vi "Cal74100.vi"() -> ()   [LabVIEW 2013]
uses:
  <vilib>/Instr/_visa.llb/VISA Configure Serial Port (Instr).vi
panel:
  out "Info":string
  in  "Zero 3":string
  in  "Zero 2":string
  in  "Zero 1":string
  in  "Set":bool
  in  "Wavelength":string
  in  "Filt6":bool
  in  "Filt5":bool
  in  "Filt4":bool
  in  "Filt3":bool
  in  "Filt2":bool
  in  "Filt1":bool
  in  "Grat3":bool
  in  "Grat2":bool
  in  "Port2":bool
  in  "Port1":bool
  in  "Grat1":bool
  in  "CloseS":bool
  in  "OpenS":bool
  in  "Filter 6":string="\r\n"
  in  "Filter 5":string
  in  "Filter 1":string="\r\n"
  in  "Filter 2":string
  in  "Filter 3":string
  in  "Filter 4":string
  in  "Write":bool
  in  "Exit":bool
  in  "Read":bool
  in  "Label 3":string
  in  "Lines 3":string
  in  "Factor 3":string
  in  "Offset 3":string
  in  "Label 2":string
  in  "Lines 2":string
  in  "Factor 2":string
  in  "Offset 2":string
  in  "Offset 1":string
  in  "Factor 1":string
  in  "Lines 1":string
  in  "Label 1":string
  out "Current Grating":string
  out "State":string
  in  "Monochromator":refnum<visa-resource-name>="COM5"
  out "Next State":string
  out "error":T1
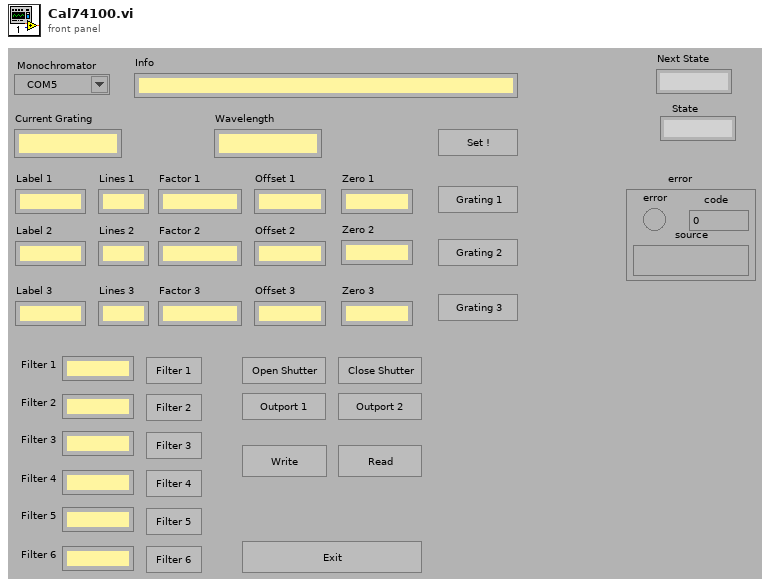
[diagram p1: front panel]
types:
  T1 = cluster{"error":bool, "code":i32, "source":string}
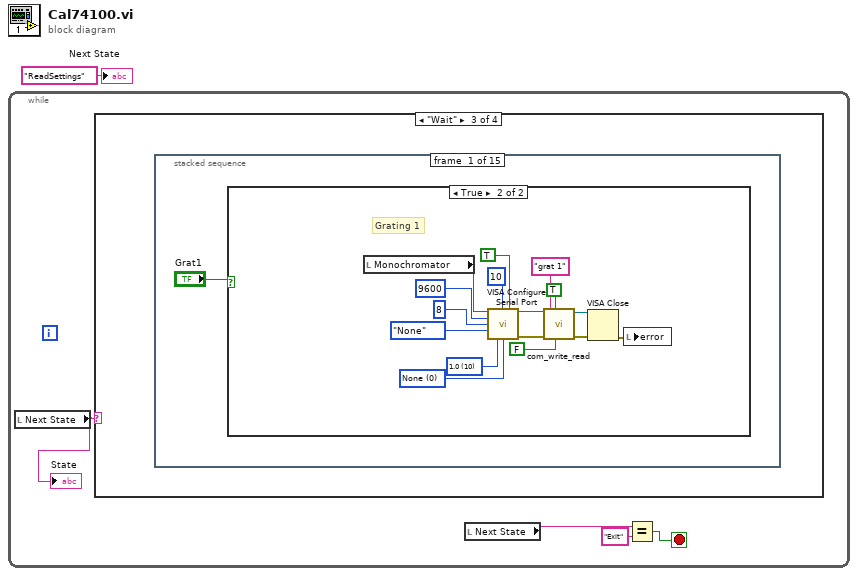
[diagram p0: block diagram]
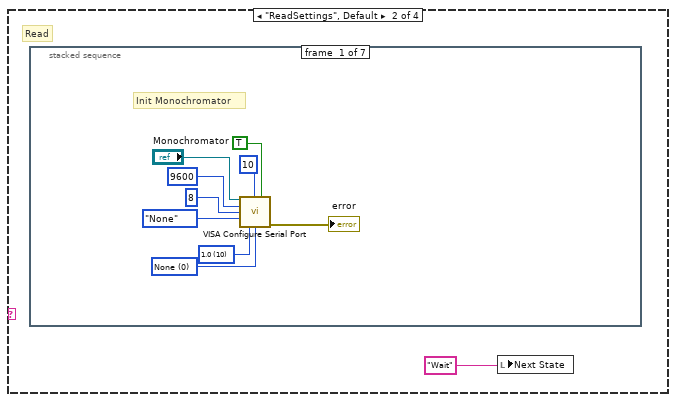
[diagram p3: hidden frame]
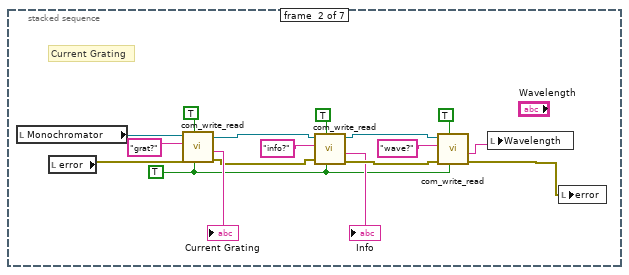
[diagram p4: hidden frame]
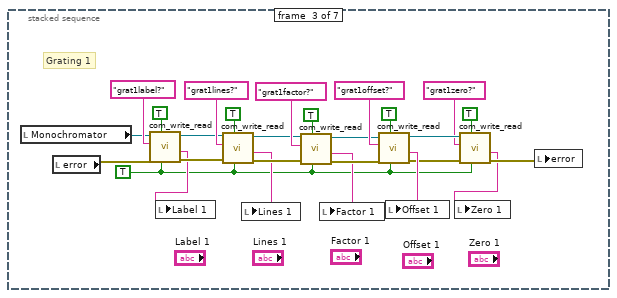
[diagram p5: hidden frame]
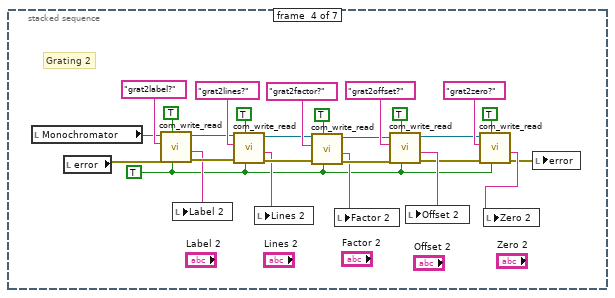
[diagram p6: hidden frame]
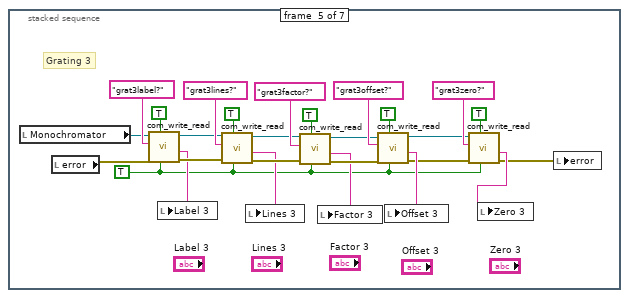
[diagram p7: hidden frame]
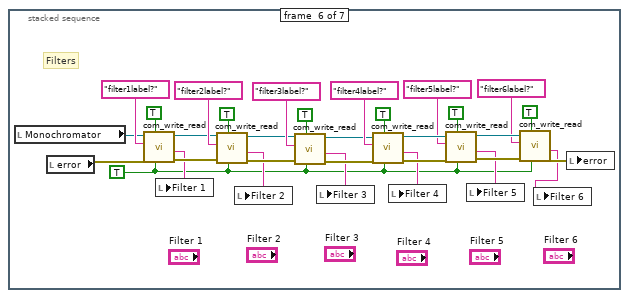
[diagram p8: hidden frame]
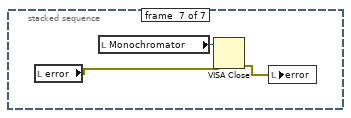
[diagram p9: hidden frame]
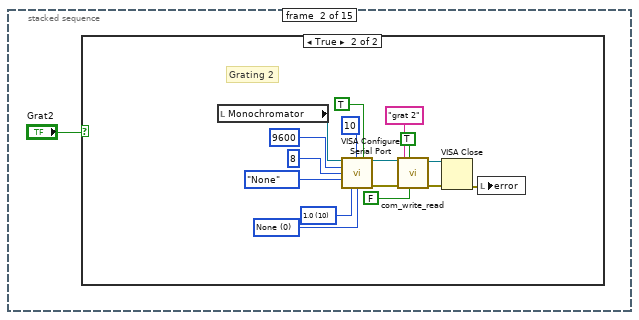
[diagram p11: hidden frame]
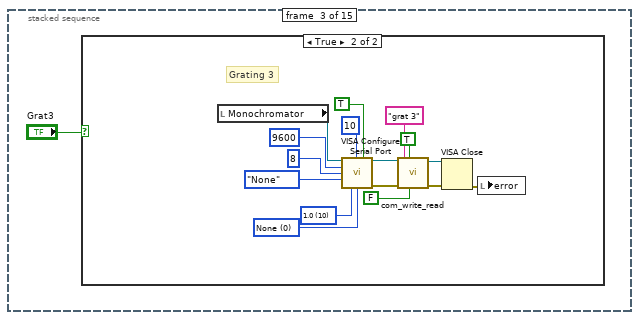
[diagram p13: hidden frame]
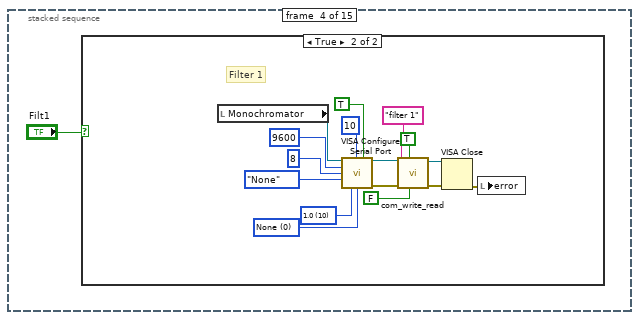
[diagram p15: hidden frame]
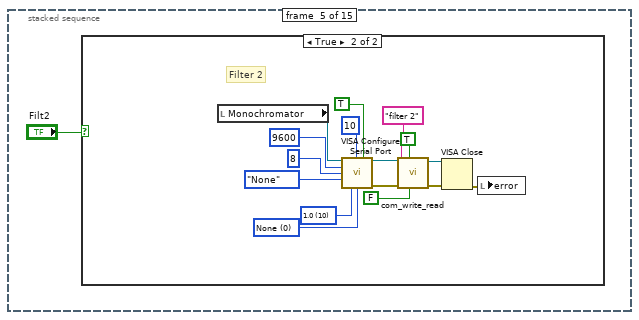
[diagram p17: hidden frame]
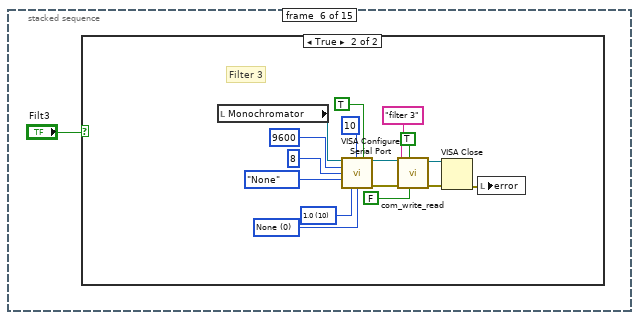
[diagram p19: hidden frame]
diagram:
  n1 = while {
    stop <- w4 stop-if-true
    n2 = local read "Next State"() -> (w2:string)
    "State" <- w2
    n3 = case shown="\"Wait\"" w2 {
      frame "Exit" {
      }
      frame "ReadSettings", Default {
        # "Read"
        n4 = stacked-sequence {
          frame #0 {
            w13 = u16 0 items=["None", "XON/XOFF", "RTS/CTS", "XON/XOFF & RTS/CTS", "DTR/DSR", "XON/XOFF & DTR/DSR"] ("flow control (0:none)")
            w12 = u16 10 items=["1.0"=10, "1.5"=15, "2.0"=20] ("stop bits (10: 1 bit)")
            # "Init Monochromator"
            n5 = call-poly "VISA Configure Serial Port"("VISA resource name"="Monochromator", "termination char\n(0xA = '\\n' = LF)"=u8 10 ("termination char\n(0xA = '\\n' = LF)"), "Enable Termination\nChar (T)"=TRUE, "baud rate (9600)"=u32 9600, "data bits (8)"=u16 8, "parity (0:none)"=enum16{"None", "Odd", "Even", "Mark", "Space"}."None", "stop bits (10: 1 bit)"=w12, "flow control (0:none)"=w13) -> ("error out"=→"error":errorcluster)  [unwired: 6 in, 1 out]
          }
          frame #1 {
            w16 = TRUE ("2 nd Query?")
            # "Current Grating"
            n6 = local read "Monochromator"() -> (w29:refnum<visa-resource-name>)
            n7 = local read "error"() -> (w30:T1)
            n8 = call "com_write_read.vi"("2 nd Query?"=w16, "Query?"=TRUE, "error in"=w30, "Command"="grat?" ("write buffer"), "VISA handle in"=w29) -> ("error out"=w21:errorcluster, "2nd Response"=→"Current Grating":string, "VISA handle out"=w20:refnum<visa-resource-name>)  [unwired: 1 in, 2 out]
            n9 = call "com_write_read.vi"("2 nd Query?"=w16, "Query?"=TRUE, "error in"=w21, "Command"="info?" ("write buffer"), "VISA handle in"=w20) -> ("error out"=w18:errorcluster, "2nd Response"=→"Info":string, "VISA handle out"=w19:refnum<visa-resource-name>)  [unwired: 1 in, 2 out]
            n10 = call "com_write_read.vi"("2 nd Query?"=w16, "Query?"=TRUE, "error in"=w18, "Command"="wave?" ("write buffer"), "VISA handle in"=w19) -> ("error out"=w26:errorcluster, "2nd Response"=w24:string)  [unwired: 1 in, 3 out]
            n11 = local write "Wavelength"(w24) -> ()
            n12 = local write "error"(w26) -> ()
          }
          frame #2 {
            w33 = TRUE ("2 nd Query?")
            # "Grating 1"
            n13 = local read "Monochromator"() -> (w56:refnum<visa-resource-name>)
            n14 = local read "error"() -> (w57:T1)
            n15 = call "com_write_read.vi"("2 nd Query?"=w33, "Query?"=TRUE, "error in"=w57, "Command"="grat1label?" ("write buffer"), "VISA handle in"=w56) -> ("error out"=w46:errorcluster, "2nd Response"=w43:string, "VISA handle out"=w49:refnum<visa-resource-name>)  [unwired: 1 in, 2 out]
            n16 = local write "Label 1"(w43) -> ()
            n17 = call "com_write_read.vi"("2 nd Query?"=w33, "Query?"=TRUE, "error in"=w46, "Command"="grat1lines?" ("write buffer"), "VISA handle in"=w49) -> ("error out"=w45:errorcluster, "2nd Response"=w42:string, "VISA handle out"=w48:refnum<visa-resource-name>)  [unwired: 1 in, 2 out]
            n18 = local write "Lines 1"(w42) -> ()
            n19 = call "com_write_read.vi"("2 nd Query?"=w33, "Query?"=TRUE, "error in"=w45, "Command"="grat1factor?" ("write buffer"), "VISA handle in"=w48) -> ("error out"=w44:errorcluster, "2nd Response"=w41:string, "VISA handle out"=w47:refnum<visa-resource-name>)  [unwired: 1 in, 2 out]
            n20 = local write "Factor 1"(w41) -> ()
            n21 = call "com_write_read.vi"("2 nd Query?"=w33, "Query?"=TRUE, "error in"=w44, "Command"="grat1offset?" ("write buffer"), "VISA handle in"=w47) -> ("error out"=w37:errorcluster, "2nd Response"=w40:string, "VISA handle out"=w38:refnum<visa-resource-name>)  [unwired: 1 in, 2 out]
            n22 = local write "Offset 1"(w40) -> ()
            n23 = call "com_write_read.vi"("2 nd Query?"=w33, "Query?"=TRUE, "error in"=w37, "Command"="grat1zero?" ("write buffer"), "VISA handle in"=w38) -> ("error out"=w36:errorcluster, "2nd Response"=w35:string)  [unwired: 1 in, 3 out]
            n24 = local write "Zero 1"(w35) -> ()
            n25 = local write "error"(w36) -> ()
          }
          frame #3 {
            w60 = TRUE ("2 nd Query?")
            # "Grating 2"
            n26 = local read "Monochromator"() -> (w83:refnum<visa-resource-name>)
            n27 = local read "error"() -> (w84:T1)
            n28 = call "com_write_read.vi"("2 nd Query?"=w60, "Query?"=TRUE, "error in"=w84, "Command"="grat2label?" ("write buffer"), "VISA handle in"=w83) -> ("error out"=w73:errorcluster, "2nd Response"=w70:string, "VISA handle out"=w76:refnum<visa-resource-name>)  [unwired: 1 in, 2 out]
            n29 = local write "Label 2"(w70) -> ()
            n30 = call "com_write_read.vi"("2 nd Query?"=w60, "Query?"=TRUE, "error in"=w73, "Command"="grat2lines?" ("write buffer"), "VISA handle in"=w76) -> ("error out"=w72:errorcluster, "2nd Response"=w69:string, "VISA handle out"=w75:refnum<visa-resource-name>)  [unwired: 1 in, 2 out]
            n31 = local write "Lines 2"(w69) -> ()
            n32 = call "com_write_read.vi"("2 nd Query?"=w60, "Query?"=TRUE, "error in"=w72, "Command"="grat2factor?" ("write buffer"), "VISA handle in"=w75) -> ("error out"=w71:errorcluster, "2nd Response"=w68:string, "VISA handle out"=w74:refnum<visa-resource-name>)  [unwired: 1 in, 2 out]
            n33 = local write "Factor 2"(w68) -> ()
            n34 = call "com_write_read.vi"("2 nd Query?"=w60, "Query?"=TRUE, "error in"=w71, "Command"="grat2offset?" ("write buffer"), "VISA handle in"=w74) -> ("error out"=w63:errorcluster, "2nd Response"=w67:string, "VISA handle out"=w64:refnum<visa-resource-name>)  [unwired: 1 in, 2 out]
            n35 = local write "Offset 2"(w67) -> ()
            n36 = call "com_write_read.vi"("2 nd Query?"=w60, "Query?"=TRUE, "error in"=w63, "Command"="grat2zero?" ("write buffer"), "VISA handle in"=w64) -> ("error out"=w61:errorcluster, "2nd Response"=w62:string)  [unwired: 1 in, 3 out]
            n37 = local write "Zero 2"(w62) -> ()
            n38 = local write "error"(w61) -> ()
          }
          frame #4 {
            w87 = TRUE ("2 nd Query?")
            # "Grating 3"
            n39 = local read "Monochromator"() -> (w110:refnum<visa-resource-name>)
            n40 = local read "error"() -> (w111:T1)
            n41 = call "com_write_read.vi"("2 nd Query?"=w87, "Query?"=TRUE, "error in"=w111, "Command"="grat3label?" ("write buffer"), "VISA handle in"=w110) -> ("error out"=w100:errorcluster, "2nd Response"=w97:string, "VISA handle out"=w103:refnum<visa-resource-name>)  [unwired: 1 in, 2 out]
            n42 = local write "Label 3"(w97) -> ()
            n43 = call "com_write_read.vi"("2 nd Query?"=w87, "Query?"=TRUE, "error in"=w100, "Command"="grat3lines?" ("write buffer"), "VISA handle in"=w103) -> ("error out"=w99:errorcluster, "2nd Response"=w96:string, "VISA handle out"=w102:refnum<visa-resource-name>)  [unwired: 1 in, 2 out]
            n44 = local write "Lines 3"(w96) -> ()
            n45 = call "com_write_read.vi"("2 nd Query?"=w87, "Query?"=TRUE, "error in"=w99, "Command"="grat3factor?" ("write buffer"), "VISA handle in"=w102) -> ("error out"=w98:errorcluster, "2nd Response"=w95:string, "VISA handle out"=w101:refnum<visa-resource-name>)  [unwired: 1 in, 2 out]
            n46 = local write "Factor 3"(w95) -> ()
            n47 = call "com_write_read.vi"("2 nd Query?"=w87, "Query?"=TRUE, "error in"=w98, "Command"="grat3offset?" ("write buffer"), "VISA handle in"=w101) -> ("error out"=w90:errorcluster, "2nd Response"=w94:string, "VISA handle out"=w91:refnum<visa-resource-name>)  [unwired: 1 in, 2 out]
            n48 = local write "Offset 3"(w94) -> ()
            n49 = call "com_write_read.vi"("2 nd Query?"=w87, "Query?"=TRUE, "error in"=w90, "Command"="grat3zero?" ("write buffer"), "VISA handle in"=w91) -> ("error out"=w88:errorcluster, "2nd Response"=w89:string)  [unwired: 1 in, 3 out]
            n50 = local write "Zero 3"(w89) -> ()
            n51 = local write "error"(w88) -> ()
          }
          frame #5 {
            w114 = TRUE ("2 nd Query?")
            # "Filters"
            n52 = local read "Monochromator"() -> (w142:refnum<visa-resource-name>)
            n53 = local read "error"() -> (w143:T1)
            n54 = call "com_write_read.vi"("2 nd Query?"=w114, "Query?"=TRUE, "error in"=w143, "Command"="filter1label?" ("write buffer"), "VISA handle in"=w142) -> ("error out"=w132:errorcluster, "2nd Response"=w115:string, "VISA handle out"=w135:refnum<visa-resource-name>)  [unwired: 1 in, 2 out]
            n55 = local write "Filter 1"(w115) -> ()
            n56 = call "com_write_read.vi"("2 nd Query?"=w114, "Query?"=TRUE, "error in"=w132, "Command"="filter2label?" ("write buffer"), "VISA handle in"=w135) -> ("error out"=w131:errorcluster, "2nd Response"=w116:string, "VISA handle out"=w134:refnum<visa-resource-name>)  [unwired: 1 in, 2 out]
            n57 = local write "Filter 2"(w116) -> ()
            n58 = call "com_write_read.vi"("2 nd Query?"=w114, "Query?"=TRUE, "error in"=w131, "Command"="filter3label?" ("write buffer"), "VISA handle in"=w134) -> ("error out"=w130:errorcluster, "2nd Response"=w117:string, "VISA handle out"=w133:refnum<visa-resource-name>)  [unwired: 1 in, 2 out]
            n59 = local write "Filter 3"(w117) -> ()
            n60 = call "com_write_read.vi"("2 nd Query?"=w114, "Query?"=TRUE, "error in"=w130, "Command"="filter4label?" ("write buffer"), "VISA handle in"=w133) -> ("error out"=w127:errorcluster, "2nd Response"=w118:string, "VISA handle out"=w124:refnum<visa-resource-name>)  [unwired: 1 in, 2 out]
            n61 = local write "Filter 4"(w118) -> ()
            n62 = call "com_write_read.vi"("2 nd Query?"=w114, "Query?"=TRUE, "error in"=w127, "Command"="filter5label?" ("write buffer"), "VISA handle in"=w124) -> ("error out"=w126:errorcluster, "2nd Response"=w119:string, "VISA handle out"=w123:refnum<visa-resource-name>)  [unwired: 1 in, 2 out]
            n63 = local write "Filter 5"(w119) -> ()
            n64 = call "com_write_read.vi"("2 nd Query?"=w114, "Query?"=TRUE, "error in"=w126, "Command"="filter6label?" ("write buffer"), "VISA handle in"=w123) -> ("error out"=w125:errorcluster, "2nd Response"=w120:string)  [unwired: 1 in, 3 out]
            n65 = local write "Filter 6"(w120) -> ()
            n66 = local write "error"(w125) -> ()
          }
          frame #6 {
            n67 = local read "error"() -> (w146:T1)
            n68 = local read "Monochromator"() -> (w148:refnum<visa-resource-name>)
            n69 = VISA Close(VISA resource name=w148, error in (no error)=w146) -> (error out=w147:errorcluster)
            n70 = local write "error"(w147) -> ()
          }
        }
        n71 = local write "Next State"("Wait") -> ()
      }
      frame "Wait" {
        n72 = stacked-sequence {
          frame #0 {
            n73 = case shown="True" "Grat1" {
              frame False {
              }
              frame True {
                w153 = u16 0 items=["None", "XON/XOFF", "RTS/CTS", "XON/XOFF & RTS/CTS", "DTR/DSR", "XON/XOFF & DTR/DSR"] ("flow control (0:none)")
                w154 = u16 10 items=["1.0"=10, "1.5"=15, "2.0"=20] ("stop bits (10: 1 bit)")
                # "Grating 1"
                n74 = local read "Monochromator"() -> (w158:refnum<visa-resource-name>)
                n75 = call-poly "VISA Configure Serial Port"("VISA resource name"=w158, "termination char\n(0xA = '\\n' = LF)"=u8 10 ("termination char\n(0xA = '\\n' = LF)"), "Enable Termination\nChar (T)"=TRUE, "baud rate (9600)"=u32 9600, "data bits (8)"=u16 8, "parity (0:none)"=enum16{"None", "Odd", "Even", "Mark", "Space"}."None", "stop bits (10: 1 bit)"=w154, "flow control (0:none)"=w153) -> ("VISA resource name out"=w163:refnum<visa-resource-name>, "error out"=w162:errorcluster)  [unwired: 6 in]
                n76 = call "com_write_read.vi"("2 nd Query?"=FALSE, "Query?"=TRUE, "error in"=w162, "Command"="grat 1" ("write buffer"), "VISA handle in"=w163) -> ("error out"=w165:errorcluster, "VISA handle out"=w164:refnum<visa-resource-name>)  [unwired: 1 in, 3 out]
                n77 = VISA Close(VISA resource name=w164, error in (no error)=w165) -> (error out=w159:errorcluster)
                n78 = local write "error"(w159) -> ()
              }
            }
          }
          frame #1 {
            n79 = case shown="True" "Grat2" {
              frame False {
              }
              frame True {
                w170 = u16 0 items=["None", "XON/XOFF", "RTS/CTS", "XON/XOFF & RTS/CTS", "DTR/DSR", "XON/XOFF & DTR/DSR"] ("flow control (0:none)")
                w171 = u16 10 items=["1.0"=10, "1.5"=15, "2.0"=20] ("stop bits (10: 1 bit)")
                # "Grating 2"
                n80 = local read "Monochromator"() -> (w175:refnum<visa-resource-name>)
                n81 = call-poly "VISA Configure Serial Port"("VISA resource name"=w175, "termination char\n(0xA = '\\n' = LF)"=u8 10 ("termination char\n(0xA = '\\n' = LF)"), "Enable Termination\nChar (T)"=TRUE, "baud rate (9600)"=u32 9600, "data bits (8)"=u16 8, "parity (0:none)"=enum16{"None", "Odd", "Even", "Mark", "Space"}."None", "stop bits (10: 1 bit)"=w171, "flow control (0:none)"=w170) -> ("VISA resource name out"=w180:refnum<visa-resource-name>, "error out"=w179:errorcluster)  [unwired: 6 in]
                n82 = call "com_write_read.vi"("2 nd Query?"=FALSE, "Query?"=TRUE, "error in"=w179, "Command"="grat 2" ("write buffer"), "VISA handle in"=w180) -> ("error out"=w182:errorcluster, "VISA handle out"=w181:refnum<visa-resource-name>)  [unwired: 1 in, 3 out]
                n83 = VISA Close(VISA resource name=w181, error in (no error)=w182) -> (error out=w176:errorcluster)
                n84 = local write "error"(w176) -> ()
              }
            }
          }
          frame #2 {
            n85 = case shown="True" "Grat3" {
              frame False {
              }
              frame True {
                w187 = u16 0 items=["None", "XON/XOFF", "RTS/CTS", "XON/XOFF & RTS/CTS", "DTR/DSR", "XON/XOFF & DTR/DSR"] ("flow control (0:none)")
                w188 = u16 10 items=["1.0"=10, "1.5"=15, "2.0"=20] ("stop bits (10: 1 bit)")
                # "Grating 3"
                n86 = local read "Monochromator"() -> (w192:refnum<visa-resource-name>)
                n87 = call-poly "VISA Configure Serial Port"("VISA resource name"=w192, "termination char\n(0xA = '\\n' = LF)"=u8 10 ("termination char\n(0xA = '\\n' = LF)"), "Enable Termination\nChar (T)"=TRUE, "baud rate (9600)"=u32 9600, "data bits (8)"=u16 8, "parity (0:none)"=enum16{"None", "Odd", "Even", "Mark", "Space"}."None", "stop bits (10: 1 bit)"=w188, "flow control (0:none)"=w187) -> ("VISA resource name out"=w197:refnum<visa-resource-name>, "error out"=w196:errorcluster)  [unwired: 6 in]
                n88 = call "com_write_read.vi"("2 nd Query?"=FALSE, "Query?"=TRUE, "error in"=w196, "Command"="grat 3" ("write buffer"), "VISA handle in"=w197) -> ("error out"=w199:errorcluster, "VISA handle out"=w198:refnum<visa-resource-name>)  [unwired: 1 in, 3 out]
                n89 = VISA Close(VISA resource name=w198, error in (no error)=w199) -> (error out=w193:errorcluster)
                n90 = local write "error"(w193) -> ()
              }
            }
          }
          frame #3 {
            n91 = case shown="True" "Filt1" {
              frame False {
              }
              frame True {
                w204 = u16 0 items=["None", "XON/XOFF", "RTS/CTS", "XON/XOFF & RTS/CTS", "DTR/DSR", "XON/XOFF & DTR/DSR"] ("flow control (0:none)")
                w205 = u16 10 items=["1.0"=10, "1.5"=15, "2.0"=20] ("stop bits (10: 1 bit)")
                # "Filter 1"
                n92 = local read "Monochromator"() -> (w209:refnum<visa-resource-name>)
                n93 = call-poly "VISA Configure Serial Port"("VISA resource name"=w209, "termination char\n(0xA = '\\n' = LF)"=u8 10 ("termination char\n(0xA = '\\n' = LF)"), "Enable Termination\nChar (T)"=TRUE, "baud rate (9600)"=u32 9600, "data bits (8)"=u16 8, "parity (0:none)"=enum16{"None", "Odd", "Even", "Mark", "Space"}."None", "stop bits (10: 1 bit)"=w205, "flow control (0:none)"=w204) -> ("VISA resource name out"=w214:refnum<visa-resource-name>, "error out"=w213:errorcluster)  [unwired: 6 in]
                n94 = call "com_write_read.vi"("2 nd Query?"=FALSE, "Query?"=TRUE, "error in"=w213, "Command"="filter 1" ("write buffer"), "VISA handle in"=w214) -> ("error out"=w216:errorcluster, "VISA handle out"=w215:refnum<visa-resource-name>)  [unwired: 1 in, 3 out]
                n95 = VISA Close(VISA resource name=w215, error in (no error)=w216) -> (error out=w210:errorcluster)
                n96 = local write "error"(w210) -> ()
              }
            }
          }
          frame #4 {
            n97 = case shown="True" "Filt2" {
              frame False {
              }
              frame True {
                w221 = u16 0 items=["None", "XON/XOFF", "RTS/CTS", "XON/XOFF & RTS/CTS", "DTR/DSR", "XON/XOFF & DTR/DSR"] ("flow control (0:none)")
                w222 = u16 10 items=["1.0"=10, "1.5"=15, "2.0"=20] ("stop bits (10: 1 bit)")
                # "Filter 2"
                n98 = local read "Monochromator"() -> (w226:refnum<visa-resource-name>)
                n99 = call-poly "VISA Configure Serial Port"("VISA resource name"=w226, "termination char\n(0xA = '\\n' = LF)"=u8 10 ("termination char\n(0xA = '\\n' = LF)"), "Enable Termination\nChar (T)"=TRUE, "baud rate (9600)"=u32 9600, "data bits (8)"=u16 8, "parity (0:none)"=enum16{"None", "Odd", "Even", "Mark", "Space"}."None", "stop bits (10: 1 bit)"=w222, "flow control (0:none)"=w221) -> ("VISA resource name out"=w231:refnum<visa-resource-name>, "error out"=w230:errorcluster)  [unwired: 6 in]
                n100 = call "com_write_read.vi"("2 nd Query?"=FALSE, "Query?"=TRUE, "error in"=w230, "Command"="filter 2" ("write buffer"), "VISA handle in"=w231) -> ("error out"=w233:errorcluster, "VISA handle out"=w232:refnum<visa-resource-name>)  [unwired: 1 in, 3 out]
                n101 = VISA Close(VISA resource name=w232, error in (no error)=w233) -> (error out=w227:errorcluster)
                n102 = local write "error"(w227) -> ()
              }
            }
          }
          frame #5 {
            n103 = case shown="True" "Filt3" {
              frame False {
              }
              frame True {
                w238 = u16 0 items=["None", "XON/XOFF", "RTS/CTS", "XON/XOFF & RTS/CTS", "DTR/DSR", "XON/XOFF & DTR/DSR"] ("flow control (0:none)")
                w239 = u16 10 items=["1.0"=10, "1.5"=15, "2.0"=20] ("stop bits (10: 1 bit)")
                # "Filter 3"
                n104 = local read "Monochromator"() -> (w243:refnum<visa-resource-name>)
                n105 = call-poly "VISA Configure Serial Port"("VISA resource name"=w243, "termination char\n(0xA = '\\n' = LF)"=u8 10 ("termination char\n(0xA = '\\n' = LF)"), "Enable Termination\nChar (T)"=TRUE, "baud rate (9600)"=u32 9600, "data bits (8)"=u16 8, "parity (0:none)"=enum16{"None", "Odd", "Even", "Mark", "Space"}."None", "stop bits (10: 1 bit)"=w239, "flow control (0:none)"=w238) -> ("VISA resource name out"=w248:refnum<visa-resource-name>, "error out"=w247:errorcluster)  [unwired: 6 in]
                n106 = call "com_write_read.vi"("2 nd Query?"=FALSE, "Query?"=TRUE, "error in"=w247, "Command"="filter 3" ("write buffer"), "VISA handle in"=w248) -> ("error out"=w250:errorcluster, "VISA handle out"=w249:refnum<visa-resource-name>)  [unwired: 1 in, 3 out]
                n107 = VISA Close(VISA resource name=w249, error in (no error)=w250) -> (error out=w244:errorcluster)
                n108 = local write "error"(w244) -> ()
              }
            }
          }
          frame #6 {
            n109 = case shown="True" "Filt4" {
              frame False {
              }
              frame True {
                w255 = u16 0 items=["None", "XON/XOFF", "RTS/CTS", "XON/XOFF & RTS/CTS", "DTR/DSR", "XON/XOFF & DTR/DSR"] ("flow control (0:none)")
                w256 = u16 10 items=["1.0"=10, "1.5"=15, "2.0"=20] ("stop bits (10: 1 bit)")
                # "Filter 4"
                n110 = local read "Monochromator"() -> (w260:refnum<visa-resource-name>)
                n111 = call-poly "VISA Configure Serial Port"("VISA resource name"=w260, "termination char\n(0xA = '\\n' = LF)"=u8 10 ("termination char\n(0xA = '\\n' = LF)"), "Enable Termination\nChar (T)"=TRUE, "baud rate (9600)"=u32 9600, "data bits (8)"=u16 8, "parity (0:none)"=enum16{"None", "Odd", "Even", "Mark", "Space"}."None", "stop bits (10: 1 bit)"=w256, "flow control (0:none)"=w255) -> ("VISA resource name out"=w265:refnum<visa-resource-name>, "error out"=w264:errorcluster)  [unwired: 6 in]
                n112 = call "com_write_read.vi"("2 nd Query?"=FALSE, "Query?"=TRUE, "error in"=w264, "Command"="filter 4" ("write buffer"), "VISA handle in"=w265) -> ("error out"=w267:errorcluster, "VISA handle out"=w266:refnum<visa-resource-name>)  [unwired: 1 in, 3 out]
                n113 = VISA Close(VISA resource name=w266, error in (no error)=w267) -> (error out=w261:errorcluster)
                n114 = local write "error"(w261) -> ()
              }
            }
          }
          frame #7 {
            n115 = case shown="True" "Filt5" {
              frame False {
              }
              frame True {
                w272 = u16 0 items=["None", "XON/XOFF", "RTS/CTS", "XON/XOFF & RTS/CTS", "DTR/DSR", "XON/XOFF & DTR/DSR"] ("flow control (0:none)")
                w273 = u16 10 items=["1.0"=10, "1.5"=15, "2.0"=20] ("stop bits (10: 1 bit)")
                # "Filter5"
                n116 = local read "Monochromator"() -> (w277:refnum<visa-resource-name>)
                n117 = call-poly "VISA Configure Serial Port"("VISA resource name"=w277, "termination char\n(0xA = '\\n' = LF)"=u8 10 ("termination char\n(0xA = '\\n' = LF)"), "Enable Termination\nChar (T)"=TRUE, "baud rate (9600)"=u32 9600, "data bits (8)"=u16 8, "parity (0:none)"=enum16{"None", "Odd", "Even", "Mark", "Space"}."None", "stop bits (10: 1 bit)"=w273, "flow control (0:none)"=w272) -> ("VISA resource name out"=w282:refnum<visa-resource-name>, "error out"=w281:errorcluster)  [unwired: 6 in]
                n118 = call "com_write_read.vi"("2 nd Query?"=FALSE, "Query?"=TRUE, "error in"=w281, "Command"="filter 5" ("write buffer"), "VISA handle in"=w282) -> ("error out"=w284:errorcluster, "VISA handle out"=w283:refnum<visa-resource-name>)  [unwired: 1 in, 3 out]
                n119 = VISA Close(VISA resource name=w283, error in (no error)=w284) -> (error out=w278:errorcluster)
                n120 = local write "error"(w278) -> ()
              }
            }
          }
          frame #8 {
            n121 = case shown="True" "Filt6" {
              frame False {
              }
              frame True {
                w289 = u16 0 items=["None", "XON/XOFF", "RTS/CTS", "XON/XOFF & RTS/CTS", "DTR/DSR", "XON/XOFF & DTR/DSR"] ("flow control (0:none)")
                w290 = u16 10 items=["1.0"=10, "1.5"=15, "2.0"=20] ("stop bits (10: 1 bit)")
                # "Filter 6"
                n122 = local read "Monochromator"() -> (w294:refnum<visa-resource-name>)
                n123 = call-poly "VISA Configure Serial Port"("VISA resource name"=w294, "termination char\n(0xA = '\\n' = LF)"=u8 10 ("termination char\n(0xA = '\\n' = LF)"), "Enable Termination\nChar (T)"=TRUE, "baud rate (9600)"=u32 9600, "data bits (8)"=u16 8, "parity (0:none)"=enum16{"None", "Odd", "Even", "Mark", "Space"}."None", "stop bits (10: 1 bit)"=w290, "flow control (0:none)"=w289) -> ("VISA resource name out"=w299:refnum<visa-resource-name>, "error out"=w298:errorcluster)  [unwired: 6 in]
                n124 = call "com_write_read.vi"("2 nd Query?"=FALSE, "Query?"=TRUE, "error in"=w298, "Command"="filter 6" ("write buffer"), "VISA handle in"=w299) -> ("error out"=w301:errorcluster, "VISA handle out"=w300:refnum<visa-resource-name>)  [unwired: 1 in, 3 out]
                n125 = VISA Close(VISA resource name=w300, error in (no error)=w301) -> (error out=w295:errorcluster)
                n126 = local write "error"(w295) -> ()
              }
            }
          }
          frame #9 {
            n127 = case shown="True" "OpenS" {
              frame False {
              }
              frame True {
                w306 = u16 0 items=["None", "XON/XOFF", "RTS/CTS", "XON/XOFF & RTS/CTS", "DTR/DSR", "XON/XOFF & DTR/DSR"] ("flow control (0:none)")
                w307 = u16 10 items=["1.0"=10, "1.5"=15, "2.0"=20] ("stop bits (10: 1 bit)")
                # "OpenShutter"
                n128 = local read "Monochromator"() -> (w311:refnum<visa-resource-name>)
                n129 = call-poly "VISA Configure Serial Port"("VISA resource name"=w311, "termination char\n(0xA = '\\n' = LF)"=u8 10 ("termination char\n(0xA = '\\n' = LF)"), "Enable Termination\nChar (T)"=TRUE, "baud rate (9600)"=u32 9600, "data bits (8)"=u16 8, "parity (0:none)"=enum16{"None", "Odd", "Even", "Mark", "Space"}."None", "stop bits (10: 1 bit)"=w307, "flow control (0:none)"=w306) -> ("VISA resource name out"=w316:refnum<visa-resource-name>, "error out"=w315:errorcluster)  [unwired: 6 in]
                n130 = call "com_write_read.vi"("2 nd Query?"=FALSE, "Query?"=TRUE, "error in"=w315, "Command"="shutter o" ("write buffer"), "VISA handle in"=w316) -> ("error out"=w318:errorcluster, "VISA handle out"=w317:refnum<visa-resource-name>)  [unwired: 1 in, 3 out]
                n131 = VISA Close(VISA resource name=w317, error in (no error)=w318) -> (error out=w312:errorcluster)
                n132 = local write "error"(w312) -> ()
              }
            }
          }
          frame #10 {
            n133 = case shown="True" "CloseS" {
              frame False {
              }
              frame True {
                w323 = u16 0 items=["None", "XON/XOFF", "RTS/CTS", "XON/XOFF & RTS/CTS", "DTR/DSR", "XON/XOFF & DTR/DSR"] ("flow control (0:none)")
                w324 = u16 10 items=["1.0"=10, "1.5"=15, "2.0"=20] ("stop bits (10: 1 bit)")
                # "CloseShutter"
                n134 = local read "Monochromator"() -> (w328:refnum<visa-resource-name>)
                n135 = call-poly "VISA Configure Serial Port"("VISA resource name"=w328, "termination char\n(0xA = '\\n' = LF)"=u8 10 ("termination char\n(0xA = '\\n' = LF)"), "Enable Termination\nChar (T)"=TRUE, "baud rate (9600)"=u32 9600, "data bits (8)"=u16 8, "parity (0:none)"=enum16{"None", "Odd", "Even", "Mark", "Space"}."None", "stop bits (10: 1 bit)"=w324, "flow control (0:none)"=w323) -> ("VISA resource name out"=w333:refnum<visa-resource-name>, "error out"=w332:errorcluster)  [unwired: 6 in]
                n136 = call "com_write_read.vi"("2 nd Query?"=FALSE, "Query?"=TRUE, "error in"=w332, "Command"="shutter c" ("write buffer"), "VISA handle in"=w333) -> ("error out"=w335:errorcluster, "VISA handle out"=w334:refnum<visa-resource-name>)  [unwired: 1 in, 3 out]
                n137 = VISA Close(VISA resource name=w334, error in (no error)=w335) -> (error out=w329:errorcluster)
                n138 = local write "error"(w329) -> ()
              }
            }
          }
          frame #11 {
            n139 = case shown="True" "Port1" {
              frame False {
              }
              frame True {
                w340 = u16 0 items=["None", "XON/XOFF", "RTS/CTS", "XON/XOFF & RTS/CTS", "DTR/DSR", "XON/XOFF & DTR/DSR"] ("flow control (0:none)")
                w341 = u16 10 items=["1.0"=10, "1.5"=15, "2.0"=20] ("stop bits (10: 1 bit)")
                # "Port 1"
                n140 = local read "Monochromator"() -> (w345:refnum<visa-resource-name>)
                n141 = call-poly "VISA Configure Serial Port"("VISA resource name"=w345, "termination char\n(0xA = '\\n' = LF)"=u8 10 ("termination char\n(0xA = '\\n' = LF)"), "Enable Termination\nChar (T)"=TRUE, "baud rate (9600)"=u32 9600, "data bits (8)"=u16 8, "parity (0:none)"=enum16{"None", "Odd", "Even", "Mark", "Space"}."None", "stop bits (10: 1 bit)"=w341, "flow control (0:none)"=w340) -> ("VISA resource name out"=w350:refnum<visa-resource-name>, "error out"=w349:errorcluster)  [unwired: 6 in]
                n142 = call "com_write_read.vi"("2 nd Query?"=FALSE, "Query?"=TRUE, "error in"=w349, "Command"="outport 1" ("write buffer"), "VISA handle in"=w350) -> ("error out"=w352:errorcluster, "VISA handle out"=w351:refnum<visa-resource-name>)  [unwired: 1 in, 3 out]
                n143 = VISA Close(VISA resource name=w351, error in (no error)=w352) -> (error out=w346:errorcluster)
                n144 = local write "error"(w346) -> ()
              }
            }
          }
          frame #12 {
            n145 = case shown="True" "Port2" {
              frame False {
              }
              frame True {
                w357 = u16 0 items=["None", "XON/XOFF", "RTS/CTS", "XON/XOFF & RTS/CTS", "DTR/DSR", "XON/XOFF & DTR/DSR"] ("flow control (0:none)")
                w358 = u16 10 items=["1.0"=10, "1.5"=15, "2.0"=20] ("stop bits (10: 1 bit)")
                # "Port 2"
                n146 = local read "Monochromator"() -> (w362:refnum<visa-resource-name>)
                n147 = call-poly "VISA Configure Serial Port"("VISA resource name"=w362, "termination char\n(0xA = '\\n' = LF)"=u8 10 ("termination char\n(0xA = '\\n' = LF)"), "Enable Termination\nChar (T)"=TRUE, "baud rate (9600)"=u32 9600, "data bits (8)"=u16 8, "parity (0:none)"=enum16{"None", "Odd", "Even", "Mark", "Space"}."None", "stop bits (10: 1 bit)"=w358, "flow control (0:none)"=w357) -> ("VISA resource name out"=w367:refnum<visa-resource-name>, "error out"=w366:errorcluster)  [unwired: 6 in]
                n148 = call "com_write_read.vi"("2 nd Query?"=FALSE, "Query?"=TRUE, "error in"=w366, "Command"="outport 2" ("write buffer"), "VISA handle in"=w367) -> ("error out"=w369:errorcluster, "VISA handle out"=w368:refnum<visa-resource-name>)  [unwired: 1 in, 3 out]
                n149 = VISA Close(VISA resource name=w368, error in (no error)=w369) -> (error out=w363:errorcluster)
                n150 = local write "error"(w363) -> ()
              }
            }
          }
          frame #13 {
            n151 = case shown="True" "Set" {
              frame False {
              }
              frame True {
                w379 = u16 0 items=["None", "XON/XOFF", "RTS/CTS", "XON/XOFF & RTS/CTS", "DTR/DSR", "XON/XOFF & DTR/DSR"] ("flow control (0:none)")
                w380 = u16 10 items=["1.0"=10, "1.5"=15, "2.0"=20] ("stop bits (10: 1 bit)")
                # "Set Wavelength"
                n152 = local read "Monochromator"() -> (w384:refnum<visa-resource-name>)
                n153 = call-poly "VISA Configure Serial Port"("VISA resource name"=w384, "termination char\n(0xA = '\\n' = LF)"=u8 10 ("termination char\n(0xA = '\\n' = LF)"), "Enable Termination\nChar (T)"=TRUE, "baud rate (9600)"=u32 9600, "data bits (8)"=u16 8, "parity (0:none)"=enum16{"None", "Odd", "Even", "Mark", "Space"}."None", "stop bits (10: 1 bit)"=w380, "flow control (0:none)"=w379) -> ("VISA resource name out"=w388:refnum<visa-resource-name>, "error out"=w387:errorcluster)  [unwired: 6 in]
                n154 = local read "Wavelength"() -> (w373:string)
                n155 = String Subset(string=w373, length (rest)=8 ("length (rest)")) -> (substring=w376:string)  [unwired: 1 in]
                n156 = Concatenate Strings("gowave " ("write buffer"), w376) -> (w372:string)
                n157 = call "com_write_read.vi"("2 nd Query?"=FALSE, "Query?"=TRUE, "error in"=w387, "Command"=w372, "VISA handle in"=w388) -> ("error out"=w390:errorcluster, "VISA handle out"=w389:refnum<visa-resource-name>)  [unwired: 1 in, 3 out]
                n158 = VISA Close(VISA resource name=w389, error in (no error)=w390) -> (error out=w385:errorcluster)
                n159 = local write "error"(w385) -> ()
              }
            }
          }
          frame #14 {
            n160 = local read "Next State"() -> (w392:string)
            n161 = Select(t="Write", s="Write", f=w392) -> (s? t:f=w394:string)
            n162 = Select(t="Read", s="Read", f=w394) -> (s? t:f=w396:string)
            n163 = Select(t="Exit", s="Exit", f=w396) -> (s? t:f=w397:string)
            n164 = local write "Next State"(w397) -> ()
          }
        }
      }
      frame "Write" {
        # "Write"
        n165 = stacked-sequence {
          frame #0 {
            w408 = u16 0 items=["None", "XON/XOFF", "RTS/CTS", "XON/XOFF & RTS/CTS", "DTR/DSR", "XON/XOFF & DTR/DSR"] ("flow control (0:none)")
            w407 = u16 10 items=["1.0"=10, "1.5"=15, "2.0"=20] ("stop bits (10: 1 bit)")
            # "Init Monochromator"
            n166 = local read "Monochromator"() -> (w402:refnum<visa-resource-name>)
            n167 = call-poly "VISA Configure Serial Port"("VISA resource name"=w402, "termination char\n(0xA = '\\n' = LF)"=u8 10 ("termination char\n(0xA = '\\n' = LF)"), "Enable Termination\nChar (T)"=TRUE, "baud rate (9600)"=u32 9600, "data bits (8)"=u16 8, "parity (0:none)"=enum16{"None", "Odd", "Even", "Mark", "Space"}."None", "stop bits (10: 1 bit)"=w407, "flow control (0:none)"=w408) -> ("error out"=w403:errorcluster)  [unwired: 6 in, 1 out]
            n168 = local write "error"(w403) -> ()
          }
          frame #1 {
            # "Grating 1"
            n169 = local read "Monochromator"() -> (w441:refnum<visa-resource-name>)
            n170 = local read "Label 1"() -> (w427:string)
            n171 = local read "error"() -> (w442:T1)
            n172 = String Subset(string=w427, length (rest)=8 ("length (rest)")) -> (substring=w430:string)  [unwired: 1 in]
            n173 = Concatenate Strings("grat1label " ("write buffer"), w430) -> (w414:string)
            n174 = local read "Offset 1"() -> (w426:string)
            n175 = call "com_write_read.vi"("Query?"=TRUE, "error in"=w442, "Command"=w414, "VISA handle in"=w441) -> ("error out"=w434:errorcluster, "VISA handle out"=w437:refnum<visa-resource-name>)  [unwired: 2 in, 3 out]
            n176 = String Subset(string=w426, length (rest)=8 ("length (rest)")) -> (substring=w423:string)  [unwired: 1 in]
            n177 = Concatenate Strings("grat1offset " ("write buffer"), w423) -> (w413:string)
            n178 = local read "Lines 1"() -> (w422:string)
            n179 = call "com_write_read.vi"("Query?"=TRUE, "error in"=w434, "Command"=w413, "VISA handle in"=w437) -> ("error out"=w433:errorcluster, "VISA handle out"=w436:refnum<visa-resource-name>)  [unwired: 2 in, 3 out]
            n180 = String Subset(string=w422, length (rest)=8 ("length (rest)")) -> (substring=w419:string)  [unwired: 1 in]
            n181 = Concatenate Strings("grat1lines " ("write buffer"), w419) -> (w412:string)
            n182 = local read "Factor 1"() -> (w418:string)
            n183 = call "com_write_read.vi"("Query?"=TRUE, "error in"=w433, "Command"=w412, "VISA handle in"=w436) -> ("error out"=w432:errorcluster, "VISA handle out"=w435:refnum<visa-resource-name>)  [unwired: 2 in, 3 out]
            n184 = String Subset(string=w418, length (rest)=8 ("length (rest)")) -> (substring=w415:string)  [unwired: 1 in]
            n185 = Concatenate Strings("grat1factor " ("write buffer"), w415) -> (w411:string)
            n186 = call "com_write_read.vi"("Query?"=TRUE, "error in"=w432, "Command"=w411, "VISA handle in"=w435) -> ("error out"=w431:errorcluster)  [unwired: 2 in, 4 out]
            n187 = local write "error"(w431) -> ()
          }
          frame #2 {
            # "Grating 2"
            n188 = local read "Monochromator"() -> (w474:refnum<visa-resource-name>)
            n189 = local read "Label 2"() -> (w460:string)
            n190 = local read "error"() -> (w475:T1)
            n191 = String Subset(string=w460, length (rest)=8 ("length (rest)")) -> (substring=w463:string)  [unwired: 1 in]
            n192 = Concatenate Strings("grat2label " ("write buffer"), w463) -> (w447:string)
            n193 = local read "Offset 2"() -> (w459:string)
            n194 = call "com_write_read.vi"("Query?"=TRUE, "error in"=w475, "Command"=w447, "VISA handle in"=w474) -> ("error out"=w467:errorcluster, "VISA handle out"=w470:refnum<visa-resource-name>)  [unwired: 2 in, 3 out]
            n195 = String Subset(string=w459, length (rest)=8 ("length (rest)")) -> (substring=w456:string)  [unwired: 1 in]
            n196 = Concatenate Strings("grat2offset " ("write buffer"), w456) -> (w446:string)
            n197 = local read "Lines 2"() -> (w455:string)
            n198 = call "com_write_read.vi"("Query?"=TRUE, "error in"=w467, "Command"=w446, "VISA handle in"=w470) -> ("error out"=w466:errorcluster, "VISA handle out"=w469:refnum<visa-resource-name>)  [unwired: 2 in, 3 out]
            n199 = String Subset(string=w455, length (rest)=8 ("length (rest)")) -> (substring=w452:string)  [unwired: 1 in]
            n200 = Concatenate Strings("grat2lines " ("write buffer"), w452) -> (w445:string)
            n201 = local read "Factor 2"() -> (w451:string)
            n202 = call "com_write_read.vi"("Query?"=TRUE, "error in"=w466, "Command"=w445, "VISA handle in"=w469) -> ("error out"=w465:errorcluster, "VISA handle out"=w468:refnum<visa-resource-name>)  [unwired: 2 in, 3 out]
            n203 = String Subset(string=w451, length (rest)=8 ("length (rest)")) -> (substring=w448:string)  [unwired: 1 in]
            n204 = Concatenate Strings("grat2factor " ("write buffer"), w448) -> (w444:string)
            n205 = call "com_write_read.vi"("Query?"=TRUE, "error in"=w465, "Command"=w444, "VISA handle in"=w468) -> ("error out"=w464:errorcluster)  [unwired: 2 in, 4 out]
            n206 = local write "error"(w464) -> ()
          }
          frame #3 {
            # "Grating 3"
            n207 = local read "Monochromator"() -> (w507:refnum<visa-resource-name>)
            n208 = local read "Label 3"() -> (w493:string)
            n209 = local read "error"() -> (w508:T1)
            n210 = String Subset(string=w493, length (rest)=8 ("length (rest)")) -> (substring=w496:string)  [unwired: 1 in]
            n211 = Concatenate Strings("grat3label " ("write buffer"), w496) -> (w480:string)
            n212 = local read "Offset 3"() -> (w492:string)
            n213 = call "com_write_read.vi"("Query?"=TRUE, "error in"=w508, "Command"=w480, "VISA handle in"=w507) -> ("error out"=w500:errorcluster, "VISA handle out"=w503:refnum<visa-resource-name>)  [unwired: 2 in, 3 out]
            n214 = String Subset(string=w492, length (rest)=8 ("length (rest)")) -> (substring=w489:string)  [unwired: 1 in]
            n215 = Concatenate Strings("grat3offset " ("write buffer"), w489) -> (w479:string)
            n216 = local read "Lines 3"() -> (w488:string)
            n217 = call "com_write_read.vi"("Query?"=TRUE, "error in"=w500, "Command"=w479, "VISA handle in"=w503) -> ("error out"=w499:errorcluster, "VISA handle out"=w502:refnum<visa-resource-name>)  [unwired: 2 in, 3 out]
            n218 = String Subset(string=w488, length (rest)=8 ("length (rest)")) -> (substring=w485:string)  [unwired: 1 in]
            n219 = Concatenate Strings("grat3lines " ("write buffer"), w485) -> (w478:string)
            n220 = local read "Factor 3"() -> (w484:string)
            n221 = call "com_write_read.vi"("Query?"=TRUE, "error in"=w499, "Command"=w478, "VISA handle in"=w502) -> ("error out"=w498:errorcluster, "VISA handle out"=w501:refnum<visa-resource-name>)  [unwired: 2 in, 3 out]
            n222 = String Subset(string=w484, length (rest)=8 ("length (rest)")) -> (substring=w481:string)  [unwired: 1 in]
            n223 = Concatenate Strings("grat3factor " ("write buffer"), w481) -> (w477:string)
            n224 = call "com_write_read.vi"("Query?"=TRUE, "error in"=w498, "Command"=w477, "VISA handle in"=w501) -> ("error out"=w497:errorcluster)  [unwired: 2 in, 4 out]
            n225 = local write "error"(w497) -> ()
          }
          frame #4 {
            # "Grating Zeros"
            n226 = local read "Monochromator"() -> (w532:refnum<visa-resource-name>)
            n227 = local read "Zero 1"() -> (w522:string)
            n228 = local read "error"() -> (w533:T1)
            n229 = String Subset(string=w522, length (rest)=8 ("length (rest)")) -> (substring=w525:string)  [unwired: 1 in]
            n230 = Concatenate Strings("grat1zero " ("write buffer"), w525) -> (w513:string)
            n231 = call "com_write_read.vi"("Query?"=TRUE, "error in"=w533, "Command"=w513, "VISA handle in"=w532) -> ("error out"=w527:errorcluster, "VISA handle out"=w529:refnum<visa-resource-name>)  [unwired: 2 in, 3 out]
            n232 = local read "Zero 2"() -> (w521:string)
            n233 = String Subset(string=w521, length (rest)=8 ("length (rest)")) -> (substring=w518:string)  [unwired: 1 in]
            n234 = Concatenate Strings("grat2zero " ("write buffer"), w518) -> (w512:string)
            n235 = local read "Zero 3"() -> (w517:string)
            n236 = call "com_write_read.vi"("Query?"=TRUE, "error in"=w527, "Command"=w512, "VISA handle in"=w529) -> ("error out"=w526:errorcluster, "VISA handle out"=w528:refnum<visa-resource-name>)  [unwired: 2 in, 3 out]
            n237 = String Subset(string=w517, length (rest)=8 ("length (rest)")) -> (substring=w514:string)  [unwired: 1 in]
            n238 = Concatenate Strings("grat3zero " ("write buffer"), w514) -> (w511:string)
            n239 = call "com_write_read.vi"("Query?"=TRUE, "error in"=w526, "Command"=w511, "VISA handle in"=w528) -> ("error out"=w510:errorcluster)  [unwired: 2 in, 4 out]
            n240 = local write "error"(w510) -> ()
          }
          frame #5 {
            # "Filters"
            n241 = local read "Monochromator"() -> (w581:refnum<visa-resource-name>)
            n242 = local read "Filter 1"() -> (w561:string)
            n243 = local read "error"() -> (w582:T1)
            n244 = local read "Filter 2"() -> (w556:string)
            n245 = String Subset(string=w561, length (rest)=8 ("length (rest)")) -> (substring=w564:string)  [unwired: 1 in]
            n246 = Concatenate Strings("filter1label " ("write buffer"), w564) -> (w560:string)
            n247 = String Subset(string=w556, length (rest)=8 ("length (rest)")) -> (substring=w559:string)  [unwired: 1 in]
            n248 = call "com_write_read.vi"("Query?"=TRUE, "error in"=w582, "Command"=w560, "VISA handle in"=w581) -> ("error out"=w574:errorcluster, "VISA handle out"=w577:refnum<visa-resource-name>)  [unwired: 2 in, 3 out]
            n249 = local read "Filter 3"() -> (w551:string)
            n250 = Concatenate Strings("filter2label " ("write buffer"), w559) -> (w555:string)
            n251 = call "com_write_read.vi"("Query?"=TRUE, "error in"=w574, "Command"=w555, "VISA handle in"=w577) -> ("error out"=w573:errorcluster, "VISA handle out"=w576:refnum<visa-resource-name>)  [unwired: 2 in, 3 out]
            n252 = String Subset(string=w551, length (rest)=8 ("length (rest)")) -> (substring=w554:string)  [unwired: 1 in]
            n253 = local read "Filter 4"() -> (w546:string)
            n254 = Concatenate Strings("filter3label " ("write buffer"), w554) -> (w550:string)
            n255 = String Subset(string=w546, length (rest)=8 ("length (rest)")) -> (substring=w549:string)  [unwired: 1 in]
            n256 = call "com_write_read.vi"("Query?"=TRUE, "error in"=w573, "Command"=w550, "VISA handle in"=w576) -> ("error out"=w572:errorcluster, "VISA handle out"=w575:refnum<visa-resource-name>)  [unwired: 2 in, 3 out]
            n257 = local read "Filter 5"() -> (w541:string)
            n258 = Concatenate Strings("filter4label " ("write buffer"), w549) -> (w545:string)
            n259 = local read "Filter 6"() -> (w536:string)
            n260 = String Subset(string=w541, length (rest)=8 ("length (rest)")) -> (substring=w544:string)  [unwired: 1 in]
            n261 = call "com_write_read.vi"("Query?"=TRUE, "error in"=w572, "Command"=w545, "VISA handle in"=w575) -> ("error out"=w569:errorcluster, "VISA handle out"=w566:refnum<visa-resource-name>)  [unwired: 2 in, 3 out]
            n262 = Concatenate Strings("filter5label " ("write buffer"), w544) -> (w540:string)
            n263 = String Subset(string=w536, length (rest)=8 ("length (rest)")) -> (substring=w539:string)  [unwired: 1 in]
            n264 = call "com_write_read.vi"("Query?"=TRUE, "error in"=w569, "Command"=w540, "VISA handle in"=w566) -> ("error out"=w568:errorcluster, "VISA handle out"=w565:refnum<visa-resource-name>)  [unwired: 2 in, 3 out]
            n265 = Concatenate Strings("filter6label " ("write buffer"), w539) -> (w535:string)
            n266 = call "com_write_read.vi"("Query?"=TRUE, "error in"=w568, "Command"=w535, "VISA handle in"=w565) -> ("error out"=w567:errorcluster)  [unwired: 2 in, 4 out]
            n267 = local write "error"(w567) -> ()
          }
          frame #6 {
            n268 = local read "error"() -> (w584:T1)
            n269 = local read "Monochromator"() -> (w586:refnum<visa-resource-name>)
            n270 = VISA Close(VISA resource name=w586, error in (no error)=w584) -> (error out=w585:errorcluster)
            n271 = local write "error"(w585) -> ()
          }
        }
        n272 = local write "Next State"("Wait") -> ()
      }
    }
    n273 = local read "Next State"() -> (w5:string)
    n274 = Equal?(x=w5, y="Exit") -> (x = y?=w4:bool)
  }
  "Next State" <- "ReadSettings"
